vi "Apply Encryption Transformation.vi"(8 "error in (no error)":errorcluster, 10 "Raw data in":u8[](array[numeric]), 11 "CryptoTransform in":refnum<k24>) -> (0 "error out":errorcluster, 2 "Encrypted data out":u8[](array[numeric]), 3 "CryptoTransform out":refnum<k24>)   [LabVIEW 2021, in "dotNET Crypto Symmetric Encryption.lvlib"]
doc: "Encrypt text using the supplied .NET CryptoTransform object."
uses:
  dotNET Crypto Symmetric Encryption.lvlib
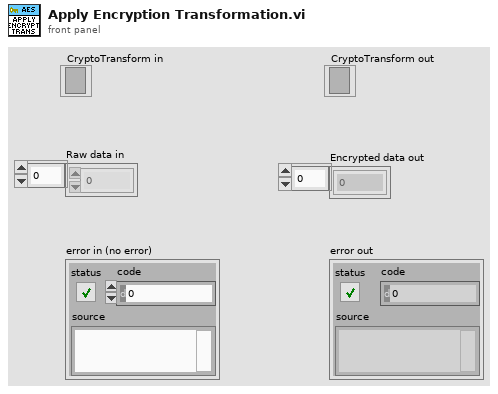
[diagram p1: front panel]
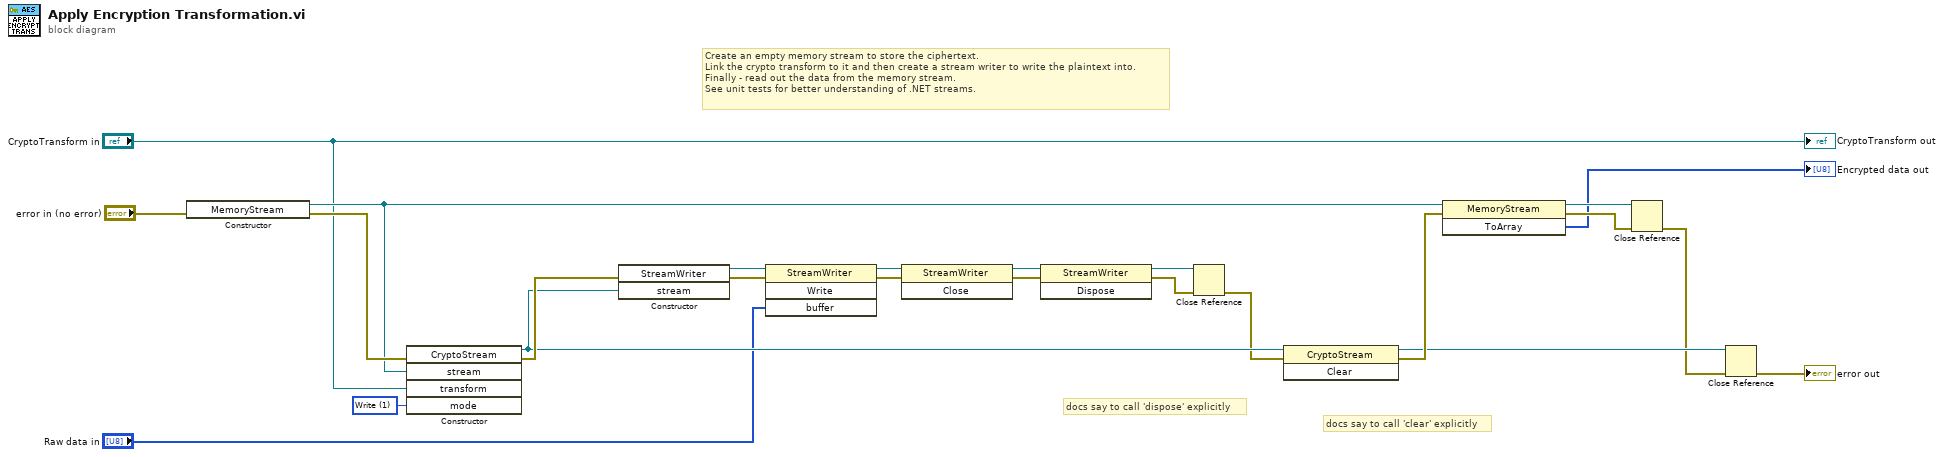
[diagram p0: block diagram]
diagram:
  w22 = 1 items=["Read", "Write"] ("mode")
  # "docs say to call 'dispose' explicitly"
  # "docs say to call 'clear' explicitly"
  # "Create an empty memory stream to store the ciphertext.\nLink the crypto transform to it and then create a stream writer to write the plaintext into.\nFinally - read out the data from the memory stream.\nSee unit tests for better understanding of .NET streams."
  n1 = constructor class="MemoryStream"(error in="error in (no error)") -> (reference out=w16:refnum<k24>, error out=w24:errorcluster)  [unwired: 2 in, 1 out]
  n2 = constructor class="CryptoStream"(error in=w24, "stream"=w16, "transform"="CryptoTransform in", "mode"=w22) -> (reference out=w15:refnum<k24>, error out=w17:errorcluster)  [unwired: 2 in, 4 out]
  n3 = constructor class="StreamWriter"(error in=w17, "stream"=w15) -> (reference out=w20:refnum<k24>, error out=w21:errorcluster)  [unwired: 2 in, 2 out]
  n4 = invoke class="StreamWriter" method="Write"(reference=w20, error in=w21, "buffer"="Raw data in") -> (reference out=w8:refnum<k24>, error out=w7:errorcluster)  [unwired: 1 in, 2 out]
  n5 = invoke class="StreamWriter" method="Close"(reference=w8, error in=w7) -> (reference out=w6:refnum<k24>, error out=w5:errorcluster)  [unwired: 1 in, 1 out]
  n6 = invoke class="StreamWriter" method="Dispose"(reference=w6, error in=w5) -> (reference out=w4:refnum<k24>, error out=w3:errorcluster)  [unwired: 1 in, 1 out]
  n7 = Close Reference(reference=w4, error in (no error)=w3) -> (error out=w2:errorcluster)
  n8 = invoke class="CryptoStream" method="Clear"(reference=w15, error in=w2) -> (reference out=w9:refnum<k24>, error out=w12:errorcluster)  [unwired: 1 in, 1 out]
  n9 = invoke class="MemoryStream" method="ToArray"(reference=w16, error in=w12) -> (reference out=w18:refnum<k24>, error out=w19:errorcluster, "ToArray"=→"Encrypted data out":u8[])  [unwired: 1 in]
  n10 = Close Reference(reference=w18, error in (no error)=w19) -> (error out=w1:errorcluster)
  n11 = Close Reference(reference=w9, error in (no error)=w1) -> (error out=→"error out":errorcluster)
  "CryptoTransform out" <- "CryptoTransform in"
